vi "Exemple_Preprocessing_PolynomialFeatures.vi"() -> ()   [LabVIEW 2020]
uses:
  Objet/6 - Datasets Transformation/6.3 - Processing Data/PolynomialFeatures/PolynomialFeatures.lvclass
panel:
  in  "y":string[][](array[string])
  in  "X":string[][](array[string])=[["0", "1"], ["2", "3"], ["4", "5"]]
  out "Data":T1
  out "error out":errorcluster
  in  "error in":errorcluster caption="entrée d'erreur"
  in  "PolynomialFeatures":T2={"degre"=2, "interaction_only"=FALSE, "include_bias"=TRUE, "order"="C"}
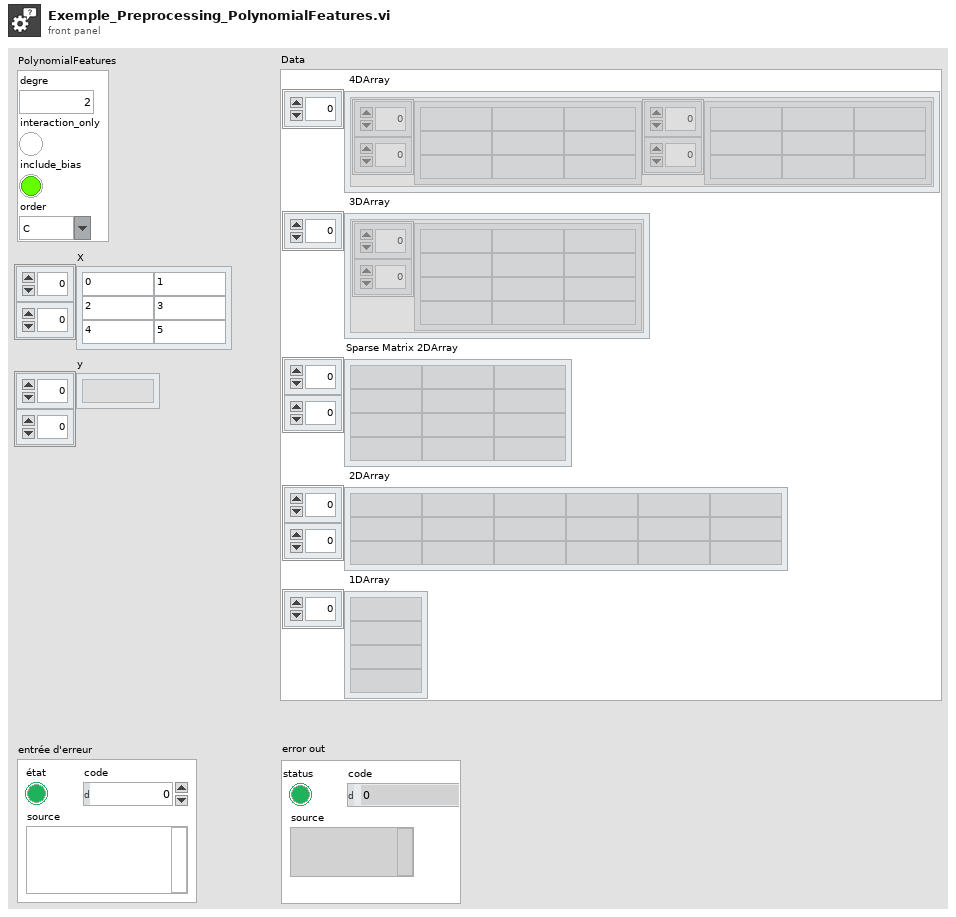
[diagram p1: front panel]
types:
  T1 = cluster{" 4DArray":cluster{"1":string[][], "2":string[][]}[], " 3DArray":cluster{"Tableau":string[][]}[], "Sparse Matrix 2DArray":string[][], " 2DArray":string[][], " 1DArray":string[]}
  T2 = cluster{"degre":i32, "interaction_only":bool, "include_bias":bool, "order":string}
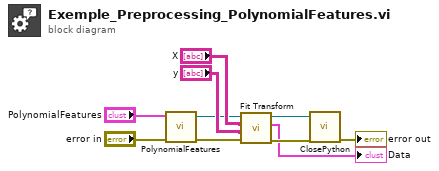
[diagram p0: block diagram]
diagram:
  n1 = call "PolynomialFeatures.vi"("error in (no error)"="error in", "PolynomialFeatures"="PolynomialFeatures") -> ("error out"=w5:errorcluster, "PolynomialFeatures.lvclass"=w7:refnum<class "PolynomialFeatures.lvclass">)  [unwired: 8 in]
  n2 = call-dynamic "Fit Transform.vi"("error in (no error)"=w5, "y"="y", "X"="X", "PolynomialFeatures.lvclass"=w7) -> ("error out"=w3:errorcluster, "Data"=→"Data":T1, "PolynomialFeatures.lvclass"=w4:refnum<class "PolynomialFeatures.lvclass">)  [unwired: 5 in]
  n3 = call-dynamic "ClosePython.vi"("error in (no error)"=w3, "Scikit-learn en entrée"=w4) -> ("error out"=→"error out":errorcluster)  [unwired: 8 in, 1 out]
